vi "SubscribedMessages.vi"() -> (3 "subscribed messages":string[](array[string]))   [LabVIEW 2017, in "OpState.lvlib"]
uses:
  <vilib>/addons/InsightCM/Devices/Shared/Common/OpState/OpState.lvlib
  <vilib>/addons/InsightCM/Devices/Shared/Common/ServerComm/ServerComm.lvlib
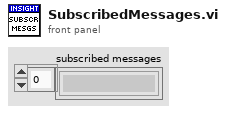
[diagram p1: front panel]
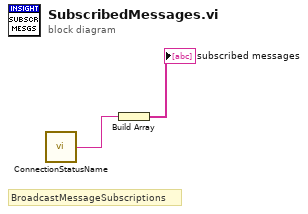
[diagram p0: block diagram]
diagram:
  # "BroadcastMessageSubscriptions"
  n1 = call <vilib>:"ConnectionStatusName.vi"() -> ("message name"=w2:string)  [unwired: 5 in]
  n2 = Build Array(w2) -> (→"subscribed messages":string[])
